vi "PH_PILS.get Status of GUI referenced Tags.vi"(2 "Tags":cluster{"GUI Ref":refnum<vi>, "Status":i32}[](array[cluster]), 3 "Tagname":string, 5 "error in":errorcluster) -> (16 "GUI Ref":refnum<vi>, 17 "Status":i32, 18 "index of element":i32, 19 "error out":errorcluster)   [LabVIEW 2014, in "PH_PILS.lvlib"]
doc: "This VI gets status, array position and GUI ref of the referenced tagname out of the array where the name is set to be the GUI ref."
uses:
  PH_PILS.lvlib
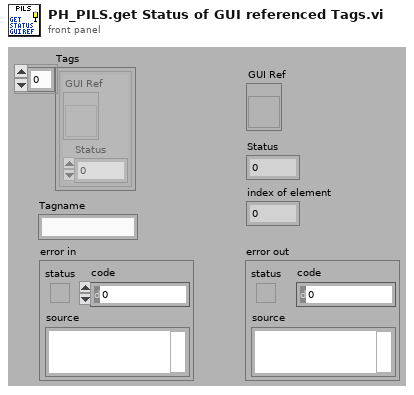
[diagram p1: front panel]
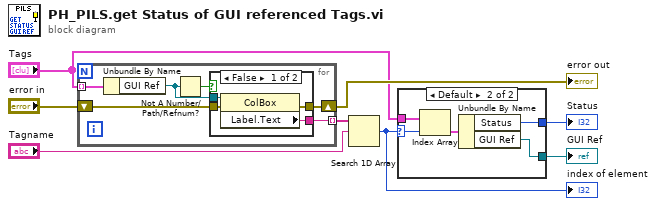
[diagram p0: block diagram]
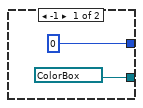
[diagram p2: hidden frame]
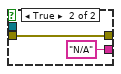
[diagram p3: hidden frame]
diagram:
  n1 = for {
    tunnel: "Tags" -> [w14] mode=indexing
    shift-right: [w10] -> w5
    shift-left: "error in" -> [w13]
    tunnel: [w9] -> w3 mode=indexing
    n2 = Unbundle By Name(w14) -> ("GUI Ref"=w11:refnum<vi>)
    n3 = Not A Number/Path/Refnum?(number/path/refnum=w11) -> (NaN/Path/Refnum?=w12:bool)
    n4 = case shown="False" w12 {
      tunnel: w11 -> [w18 _]
      tunnel: w13 -> [w17 w20]
      tunnel: [w16 w20] -> w10
      tunnel: [w15 "N/A" ("Label.Text")] -> w9
      frame False {
        n5 = property class="ColBox"(reference=w18, error in=w17) -> (error out=w16:errorcluster, "Label.Text"=w15:string)  [unwired: 1 out]
      }
      frame True {
      }
    }
  }
  "error out" <- w5
  n6 = Search 1D Array(1D array=w3, element="Tagname") -> (index of element=w7:i32)  [unwired: 1 in]
  "index of element" <- w7
  n7 = case shown="Default" w7 {
    selector: w7 -> [_ w25]
    tunnel: "Tags" -> [_ w27]
    tunnel: [0 ("Status") w24] -> w8
    tunnel: [refnum<vi> refnum ("GUI Ref") w23] -> w2
    frame -1 {
    }
    frame Default {
      n8 = Index Array(array=w27, index=w25) -> (element=w26:cluster{"GUI Ref":refnum<vi>, "Status":i32})
      n9 = Unbundle By Name(w26) -> ("Status"=w24:i32, "GUI Ref"=w23:refnum<vi>)
    }
  }
  "Status" <- w8
  "GUI Ref" <- w2
